vi "DSF.Engine.Plugin.Shutdown.vi"(8 "error in (no error)":errorcluster, 11 "Plugin in":refnum<class "DSF.Engine.Plugin.lvclass">) -> (0 "error out":errorcluster, 3 "Plugin out":refnum<class "DSF.Engine.Plugin.lvclass">)   [LabVIEW 2017, in "DSF.Engine.lvlib" / "DSF.Engine.Plugin.lvclass"]
uses:
  DSF.Engine.Plugin.lvclass
  DSF.Engine.Plugin.lvclass/DSF.Engine.Plugin.ctl
  Transceiver/DSF.Engine.Transceiver Thread.lvclass
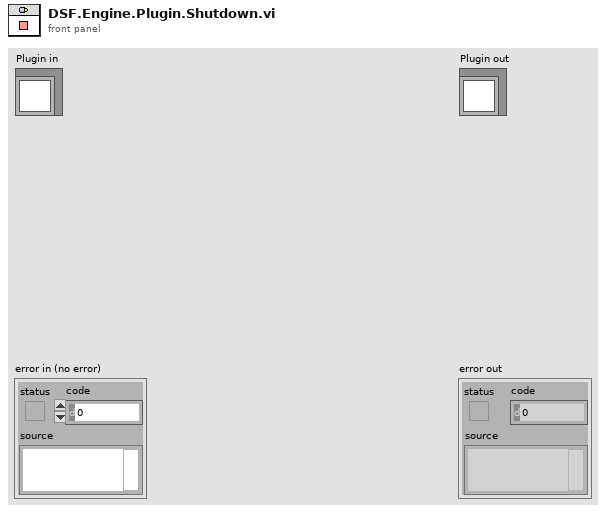
[diagram p1: front panel]
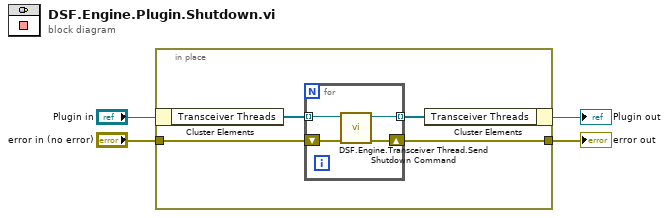
[diagram p0: block diagram]
diagram:
  n1 = in-place {
    in-place-border: "error in (no error)" -> [w8]
    in-place-border: [w7] -> w1
    n2 = in-place-cluster #1("Plugin in") -> ("Transceiver Threads"=w6:refnum<class "DSF.Engine.Interface.Transceiver.lvclass">[])
    n3 = for {
      shift-right: [w9] -> w7
      shift-left: w8 -> [w10]
      tunnel: [w11] -> w5 mode=indexing
      tunnel: w6 -> [w12] mode=indexing
      n4 = call "DSF.Engine.Transceiver Thread.Send Shutdown Command.vi"("error in (no error)"=w10, "Transceiver Interface in"=w12) -> ("error out"=w9:errorcluster, "Transceiver Interface out"=w11:refnum<class "DSF.Engine.Interface.Transceiver.lvclass">)  [unwired: 8 in]
    }
    n5 = in-place-cluster #1("Transceiver Threads"=w5) -> (→"Plugin out":refnum<class "DSF.Engine.Plugin.lvclass">)
  }
  "error out" <- w1
